vi "Kelvinox_set_zone_properties.vi"(0 "Heater_range_old":dbl, 1 "P_old":dbl, 2 "I_old":dbl, 3 "D_old":dbl, 8 "Temperature Setpoint":dbl) -> (11 "Change?":bool, 14 "Heater_range_new":dbl, 15 "P_new":dbl, 16 "I_new":dbl, 17 "D_new":dbl)   [LabVIEW 2019]
uses:
  Instrument_Setup.vi
panel:
  out "Path":path
  out "Heater table":string(combo)
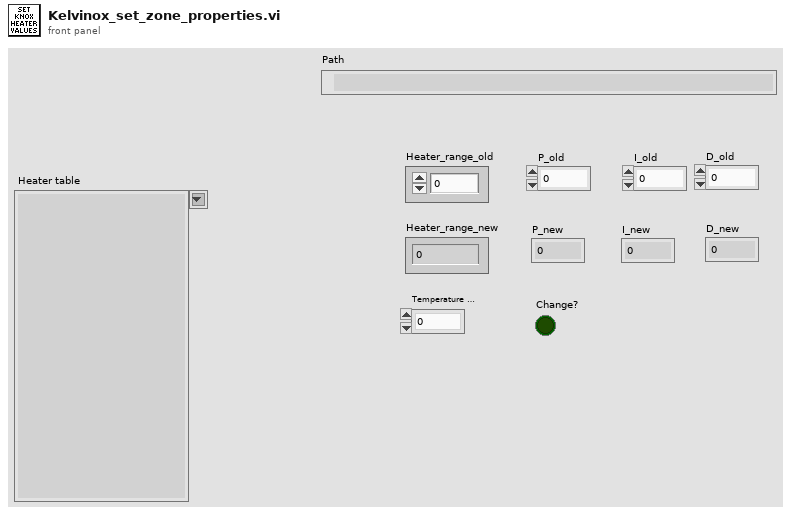
[diagram p1: front panel]
types:
  T1 = enum16{"open", "replace", "create", "open or create", "replace or create", "replace or create with confirmation"}
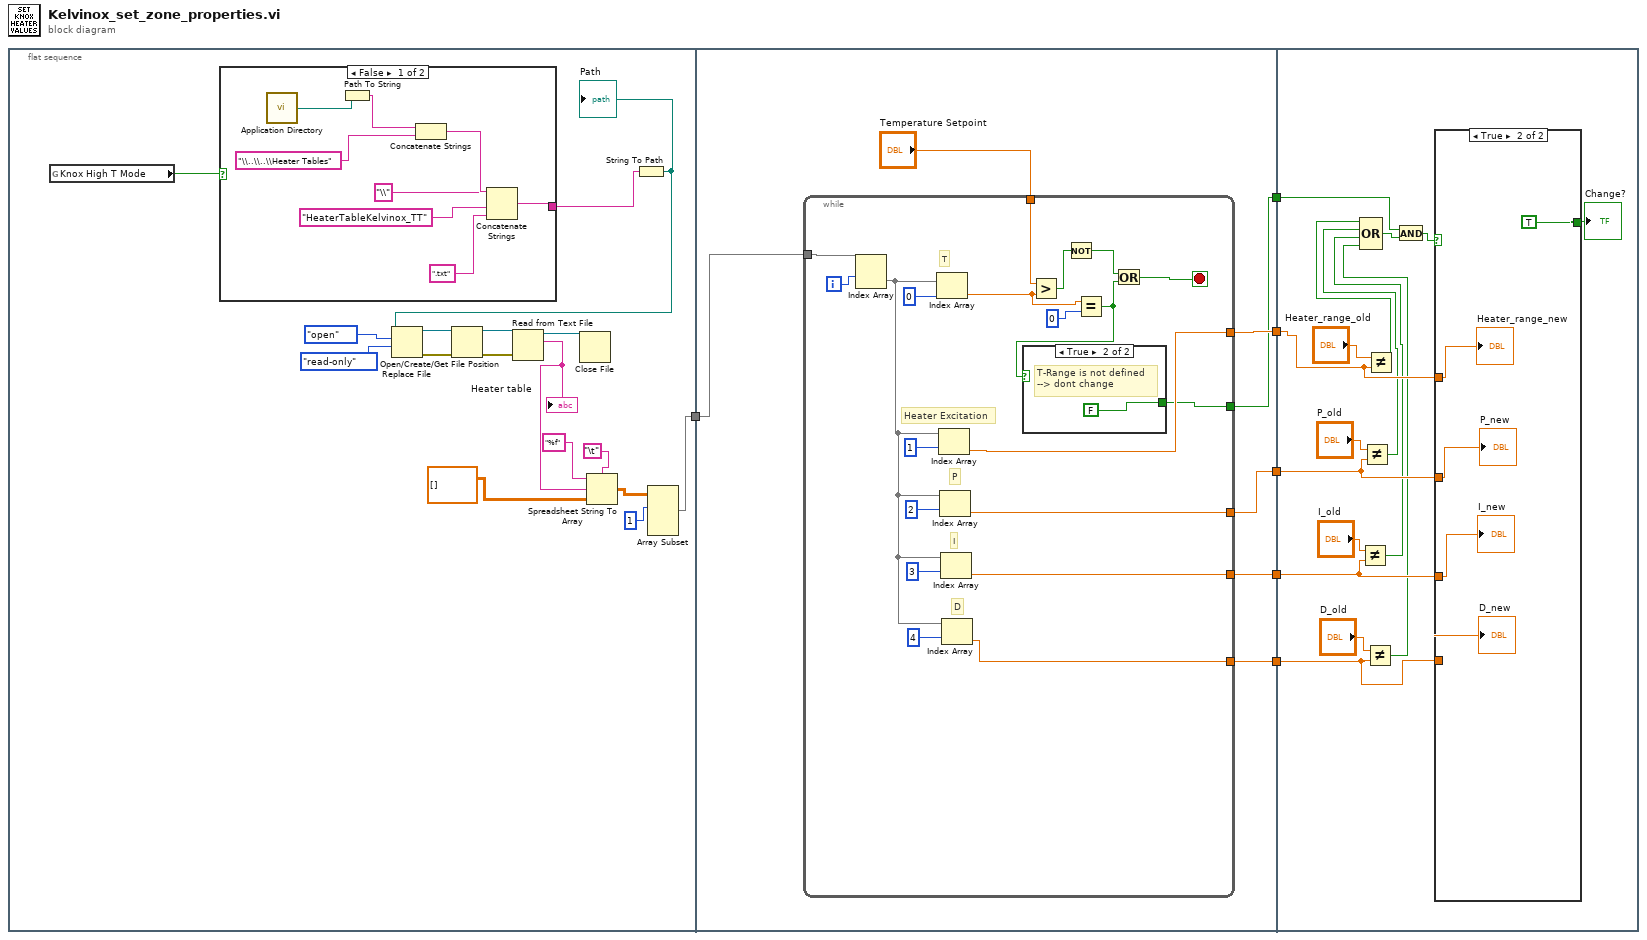
[diagram p0: block diagram]
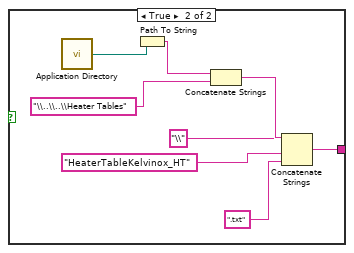
[diagram p2: hidden frame]
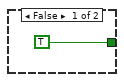
[diagram p3: hidden frame]
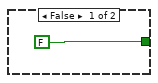
[diagram p4: hidden frame]
diagram:
  n1 = flat-sequence {
    tunnel: [w10] -> w6
    tunnel: w6 -> [w43]
    tunnel: [w46] -> w5
    tunnel: [w44] -> w4
    tunnel: [w42] -> w3
    tunnel: [w41] -> w2
    tunnel: [w40] -> w1
    tunnel: w5 -> [w82]
    tunnel: w4 -> [w71]
    tunnel: w3 -> [w78]
    tunnel: w2 -> [w77]
    tunnel: w1 -> [w76]
    frame #0 {
      n2 = global read "Instrument_Setup.vi" "Knox High T Mode"() -> (w8:bool)
      n3 = case shown="False" w8 {
        tunnel: [w24 w32] -> w7
        frame False {
          n4 = call <vilib>:"Application Directory.vi"() -> ("Application Directory"=w31:path)
          n5 = Path To String(path=w31) -> (string=w30:string)
          n6 = Concatenate Strings(w30, "\\..\\..\\Heater Tables") -> (w28:string)
          n7 = Concatenate Strings(w28, "\\", "HeaterTableKelvinox_TT", ".txt") -> (w24:string)
        }
        frame True {
          n8 = call <vilib>:"Application Directory.vi"() -> ("Application Directory"=w39:path)
          n9 = Path To String(path=w39) -> (string=w38:string)
          n10 = Concatenate Strings(w38, "\\..\\..\\Heater Tables") -> (w36:string)
          n11 = Concatenate Strings(w36, "\\", "HeaterTableKelvinox_HT", ".txt") -> (w32:string)
        }
      }
      n12 = String To Path(string=w7) -> (path=w16:path)
      "Path" <- w16
      n13 = Open/Create/Replace File(file path (use dialog)=w16, operation (0:open)=T1."open", access (0:read/write)=enum16{"read/write", "read-only", "write-only"}."read-only") -> (refnum out=w21:refnum<file>, error out=w20:errorcluster)  [unwired: 3 in, 1 out]
      n14 = Get File Position(4:w20, 7:w21) -> (0:w18:errorcluster, 3:w19:refnum<file>)  [unwired: 1 out]
      n15 = Read from Text File(file (use dialog)=w19, error in=w18) -> (refnum out=w17:refnum<file>, text=w15:string)  [unwired: 2 in, 2 out]
      "Heater table" <- w15
      n16 = Close File(refnum=w17) -> ()  [unwired: 1 in, 2 out]
      n17 = Spreadsheet String To Array(delimiter (Tab)="\t", format string="%f", spreadsheet string=w15, array type (2D Dbl)=dbl[][] []) -> (array=w11:dbl[][])
      n18 = Array Subset(array=w11, index (row)=1) -> (w10:dbl[][])  [unwired: 3 in]
    }
    frame #1 {
      n19 = while {
        tunnel: w43 -> [w66]
        tunnel: [w57] -> w46
        tunnel: "Temperature Setpoint" -> [w63]
        tunnel: [w56] -> w44
        tunnel: [w50] -> w42
        tunnel: [w49] -> w41
        tunnel: [w48] -> w40
        i -> [w55]
        stop <- w58 stop-if-true
        # "D"
        # "I"
        # "P"
        # "Heater Excitation"
        # "T"
        n20 = Index Array(array=w66, index (row)=w55) -> (element=w47:dbl[])  [unwired: 1 in]
        n21 = Index Array(array=w47, index=0) -> (element=w60:dbl)
        n22 = Index Array(array=w47, index=1) -> (element=w57:dbl)
        n23 = Index Array(array=w47, index=2) -> (element=w50:dbl)
        n24 = Index Array(array=w47, index=3) -> (element=w49:dbl)
        n25 = Index Array(array=w47, index=4) -> (element=w48:dbl)
        n26 = Greater?(x=w63, y=w60) -> (0:w62:bool)
        n27 = Not(x=w62) -> (.not. x?=w61:bool)
        n28 = Equal?(x=w60, y=0) -> (x = y?=w54:bool)
        n29 = case shown="True" w54 {
          tunnel: [TRUE FALSE] -> w56
          frame False {
          }
          frame True {
            # "T-Range is not defined\n--> dont change"
          }
        }
        n30 = Or(x=w61, y=w54) -> (x .or. y?=w58:bool)
      }
    }
    frame #2 {
      n31 = Not Equal?(x="I_old", y=w77) -> (x != y?=w73:bool)
      n32 = Not Equal?(x="P_old", y=w78) -> (x != y?=w74:bool)
      n33 = Not Equal?(x="D_old", y=w76) -> (x != y?=w72:bool)
      n34 = Not Equal?(x="Heater_range_old", y=w82) -> (x != y?=w75:bool)
      n35 = Compound Arithmetic op=OR(w75, w74, w73, w72) -> (w70:bool)
      n36 = And(x=w71, y=w70) -> (x .and. y?=w69:bool)
      n37 = case shown="True" w69 {
        tunnel: w82 -> [_ w90]
        tunnel: [FALSE TRUE] -> w84
        tunnel: w78 -> [_ w88]
        tunnel: w77 -> [_ w87]
        tunnel: w76 -> [_ w86]
        frame False {
        }
        frame True {
          "Heater_range_new" <- w90
          "P_new" <- w88
          "I_new" <- w87
          "D_new" <- w86
        }
      }
      "Change?" <- w84
    }
  }
